vi "OX Crossover Template.vi"(6 "Array Size":i32=9, 8 "Index 2":i32=5, 9 "Index 1":i32=3, 10 "Schedule 2":u16[](array[numeric]), 11 "Schedule 1":u16[](array[numeric])=[1, 3, 2, 6, 4, 5, 9, 7, 8]) -> (3 "Child":u16[](array[numeric]))   [LabVIEW 2013]
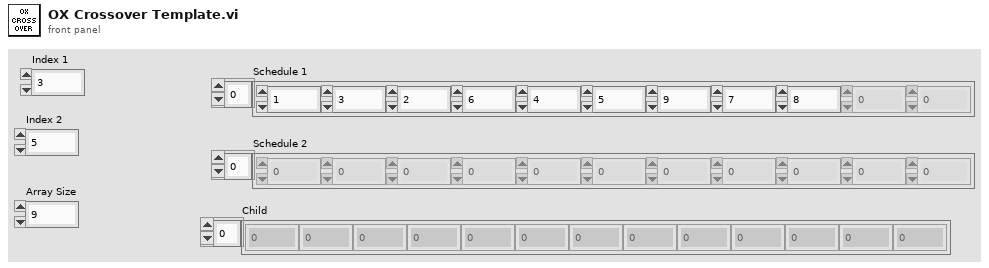
[diagram p1: front panel]
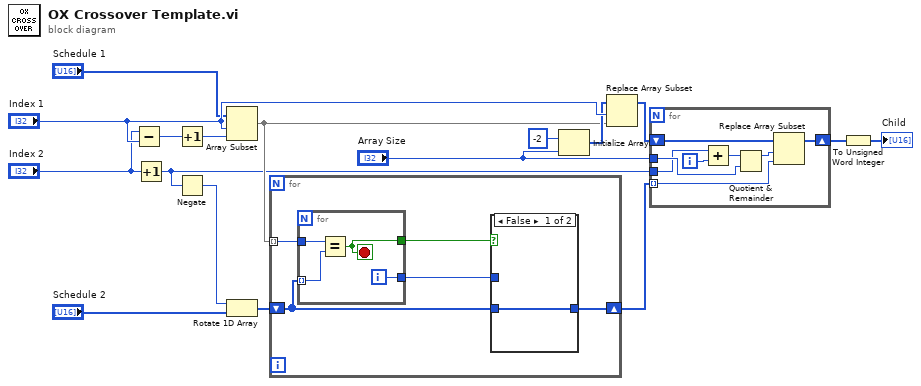
[diagram p0: block diagram]
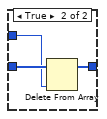
[diagram p2: hidden frame]
diagram:
  n1 = Subtract(x="Index 2", y="Index 1") -> (x-y=w12:i32)
  n2 = Increment(x="Index 2") -> (x+1=w4:i32)
  n3 = Increment(x=w12) -> (x+1=w11:i32)
  n4 = Negate(x=w4) -> (-x=w10:i32)
  n5 = Array Subset(array="Schedule 1", index="Index 1", length=w11) -> (w6:u16[])
  n6 = Rotate 1D Array(1:"Schedule 2", 2:w10) -> (0:w9:u16[])
  n7 = for {
    shift-right: [w18] -> w3
    shift-left: w9 -> [w20]
    tunnel: w6 -> [w22] mode=indexing
    n8 = for {
      tunnel: w20 -> [w29] mode=indexing
      tunnel: w22 -> [w30]
      tunnel: [w28] -> w21
      tunnel: [w27] -> w19
      i -> [w27]
      stop <- w28 stop-if-true
      n9 = Equal?(x=w30, y=w29) -> (x = y?=w28:bool)
    }
    n10 = case shown="False" w21 {
      tunnel: w20 -> [w23 w26]
      tunnel: w19 -> [_ w25]
      tunnel: [w23 w24] -> w18
      frame False {
      }
      frame True {
        n11 = Delete From Array(array=w26, index=w25) -> (array with subset deleted=w24:u16[])  [unwired: 1 in, 1 out]
      }
    }
  }
  n12 = Initialize Array(i16 -2 ("element"), "Array Size") -> (w7:i16[])
  n13 = Replace Array Subset(array=w7, new element=w6, index="Index 1") -> (w5:i16[])
  n14 = for {
    tunnel: w4 -> [w33]
    tunnel: "Array Size" -> [w38]
    tunnel: w3 -> [w35] mode=indexing
    shift-right: [w34] -> w2
    shift-left: w5 -> [w37]
    i -> [w32]
    n15 = Add(x=w33, y=w32) -> (x+y=w31:i32)
    n16 = Quotient & Remainder(x=w31, y=w38) -> (x-y*floor(x/y)=w36:i32)  [unwired: 1 out]
    n17 = Replace Array Subset(array=w37, new element=w35, index=w36) -> (w34:i16[])
  }
  n18 = To Unsigned Word Integer(number=w2) -> (unsigned 16bit integer=→"Child":u16[])
